vi "Log Time.vi"(8 "error in (no error)":errorcluster, 10 "tdms file":refnum<k34>, 11 "Acquired Result in":refnum<class "Acquired Result.lvclass">) -> (0 "error out":errorcluster, 2 "tdms file out":refnum<k34>, 3 "Acquired Result out":refnum<class "Acquired Result.lvclass">)   [LabVIEW 2019, in "Acquired Result.lvclass"]
uses:
  Acquired Result.lvclass
  Acquired Result.lvclass/Acquired Result.ctl
  Read Time group.vi
  Read Time value.vi
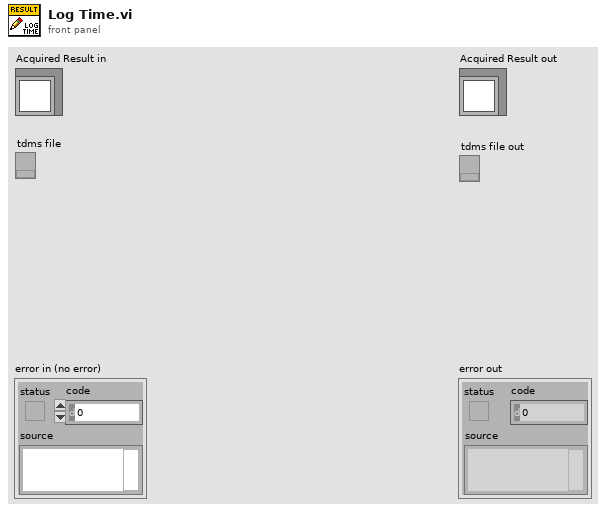
[diagram p1: front panel]
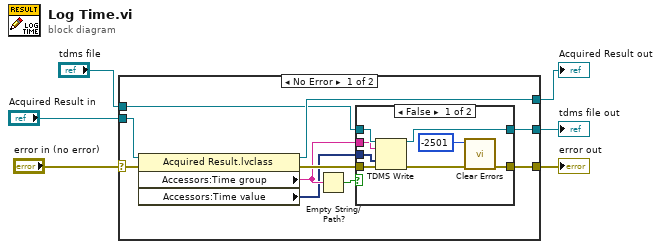
[diagram p0: block diagram]
diagram:
  n1 = case shown="No Error" "error in (no error)" {
    selector: "error in (no error)" -> [w14 w27]
    tunnel: "Acquired Result in" -> [w16 w29]
    tunnel: "tdms file" -> [w9 w28]
    tunnel: [w10 w28] -> w4
    tunnel: [w15 w29] -> w3
    tunnel: [w11 w27] -> w2
    frame No Error {
      n2 = property class="Acquired Result.lvclass"(reference=w16, error in=w14) -> (reference out=w15:refnum<class "Acquired Result.lvclass">, error out=w12:errorcluster, "Accessors:Time group"=w8:string, "Accessors:Time value"=w7:dynamicdata)
      n3 = Empty String/Path?(string/path=w8) -> (empty?=w13:bool)
      n4 = case shown="False" w13 {
        tunnel: w9 -> [w24 w26]
        tunnel: [w23 w26] -> w10
        tunnel: w8 -> [w22 _]
        tunnel: w7 -> [w21 _]
        tunnel: w12 -> [w19 w25]
        tunnel: [w18 w25] -> w11
        frame False {
          n5 = TDMS Write(0:w24, 5:w22, 9:w21, 11:w19) -> (4:w23:refnum<k34>, 15:w20:errorcluster)  [unwired: 2 in, 2 out]
          n6 = call <vilib>:"Clear Errors.vi"("error in (no error)"=w20, "specific error code to clear (0: all)"=-2501) -> ("error out"=w18:errorcluster)  [unwired: 4 in, 1 out]
        }
        frame True {
        }
      }
    }
    frame Error {
    }
  }
  "error out" <- w2
  "Acquired Result out" <- w3
  "tdms file out" <- w4
